vi "performance.vi"(1 "mSPI":u32, 2 "Loop":enum16{"Vision", "Main", "Dash"}(ring), 3 "Menu":T2) -> (0 "Performance":T1)   [LabVIEW 2014]
uses:
  typedefs/fg_getset.ctl
  typedefs/state machine/performance data.ctl
  state machine.vi
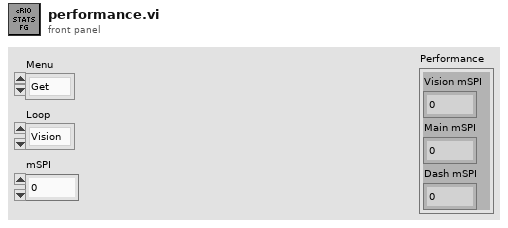
[diagram p1: front panel]
types:
  T1 = typedef "performance data.ctl" = cluster{"Vision mSPI":u32, "Main mSPI":u32, "Dash mSPI":u32}
  T2 = typedef "fg_getset.ctl" = enum16{"Get", "Set"}
  T3 = cluster{"Performance[0]":u32, "Performance[1]":u32, "Performance[2]":u32, "Performance[3]":u32, "Performance[4]":u32, "Performance[5]":u32, "Performance[6]":u32, "Performance[7]":u32, "Performance[8]":u32}
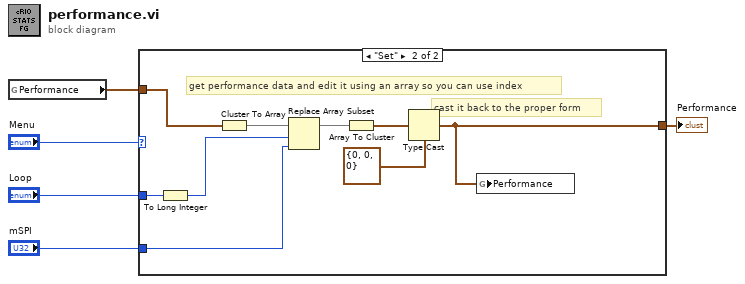
[diagram p0: block diagram]
diagram:
  n1 = global read "state machine.vi" "Performance"() -> (w1:T1)
  n2 = case shown="\"Set\"" "Menu" {
    tunnel: "Loop" -> [_ w14]
    tunnel: "mSPI" -> [_ w12]
    tunnel: [w6 w7] -> w2
    tunnel: w1 -> [w6 w8]
    frame "Get", Default {
    }
    frame "Set" {
      # "cast it back to the proper form"
      # "get performance data and edit it using an array so you can use index"
      n3 = To Long Integer(number=w14) -> (32bit integer=w13:i32)
      n4 = Cluster To Array(cluster=w8) -> (array=w15:u32[])
      n5 = Replace Array Subset(array=w15, new element=w12, index=w13) -> (w11:u32[])
      n6 = Array To Cluster(array=w11) -> (cluster=w10:T3)
      n7 = Type Cast(type=T1 {"Vision mSPI"=0, "Main mSPI"=0, "Dash mSPI"=0} ("Preformance"), x=w10) -> (*(type *) &x=w7:T1)
      n8 = global write "state machine.vi" "Performance"(w7) -> ()
    }
  }
  "Performance" <- w2
